vi "AutoFileCreatorMain.vi"() -> ()   [LabVIEW 2019]
uses:
  Utils/FilePath.vi
  <vilib>/Utility/inputDevices.llb/mouseAcquire.vi
  <vilib>/xml/NI_XML.lvlib
  <resource>/objmgr/DOMUserDefRef.rc
  <vilib>/FTP/NI_FTP.lvlib
panel:
  out "File Transfer Status":errorcluster
  in  "CopiedData":string
  in  "LocalFileNames":string[](array[string])=["1A.txt", "1B.txt", "1C.txt", "1D.txt", "2A.txt", "2B.txt", "2C.txt", "2D.txt", "3A.txt", "3B.txt", "3C.txt", "3D.txt", "4A.txt", "4B.txt", "4C.txt", "4D.txt"]
  out "standard output":string
  out "standard error":string="NI Linux Real-Time (run mode)\n\nLog in with your NI-Auth credentials.\n\n"
  in  "LocalFiles":i32(listbox)=2
  in  "SaveToLocal":bool
  in  "LoadFromLocal":bool
  in  "ExportToRobot":bool
  out "XML With IDs":string="<Sequential ID=\"1\">\n</Sequential>"
  in  "Commands":i32(listbox)=-1
  out "XML":string="<Sequential>\n</Sequential>"
  # "Instructions:\nSelect a command or structure element (Sequential, Parallel) from the Commands box and click in the XML box to the right of a \">\" to place it. \n\nAll elements in a sequential block will be executed in sequence, and those in a parallel block will be executed at the same time. You can nest these structure blocks inside themselves along with commands for complex behavior.\n\nClick ESC to unselect the current command selection.\n\nDouble click to open the options menu. Most of these options work on a specific element, but for these you do not have to click to the right of a \">\",  you can click in the element.\n\nThe Commands box is autopopulated from the VIs you put into the CommandTemplates folder in the Robot Project.\n\nYou can select a file in the LocalFiles box and load it into the editor or export it to the robot. Save your file with the save button. Make sure to save before exporting to the robot, as it exports what is saved not what is currently in the editor.\n\nNot yet implemented: Press Z to undo"
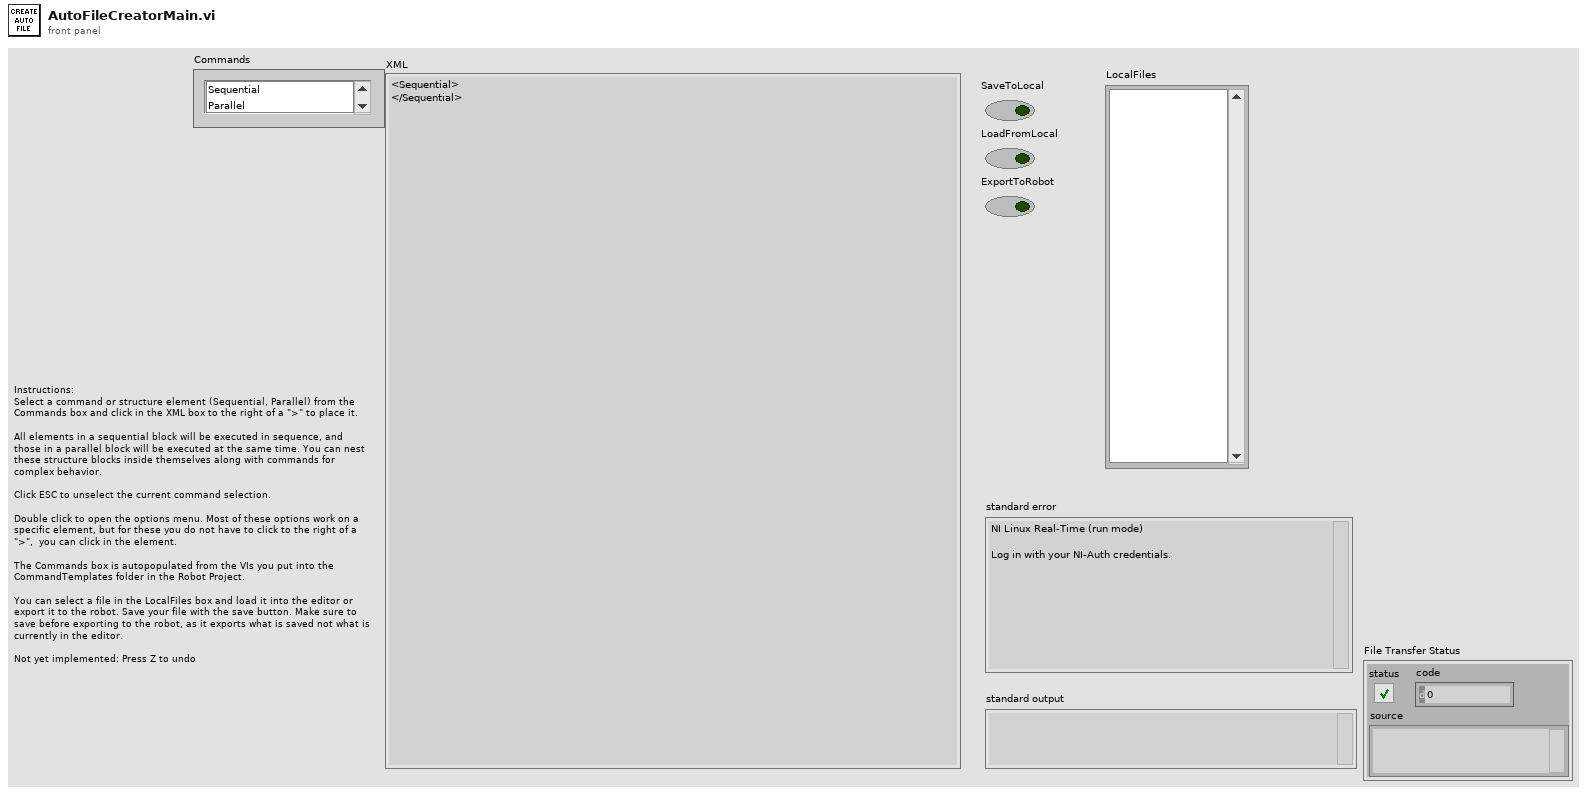
[diagram p1: front panel]
types:
  T1 = cluster{"Horizontal":i32, "Vertical":i32, "Scrolling":i32}
  T2 = typedef "eventvkey.ctl" = enum16{"ASCII", "Enter", "Return", "Shift", "Ctrl", "Alt", "Cmd", "Opt", "Caps", "NumLock", "Clear", "Break", "Up", "Down", "Left", "Right", "Insert", "Delete", "Home", "End", "PageUp", "PageDown", "Escape", "Help", "Pause", "ScrollLock", "F1", "F2", "F3", "F4", "F5", "F6", "F7", "F8", "F9", "F10", "F11", "F12", "F13", "F14", "F15", "F16", "F17", "F18", "F19", "F20", "F21", "F22", "F23", "F24", "Play", "VolumeUp", "VolumeDown", "Mute", "Two Byte Char"}
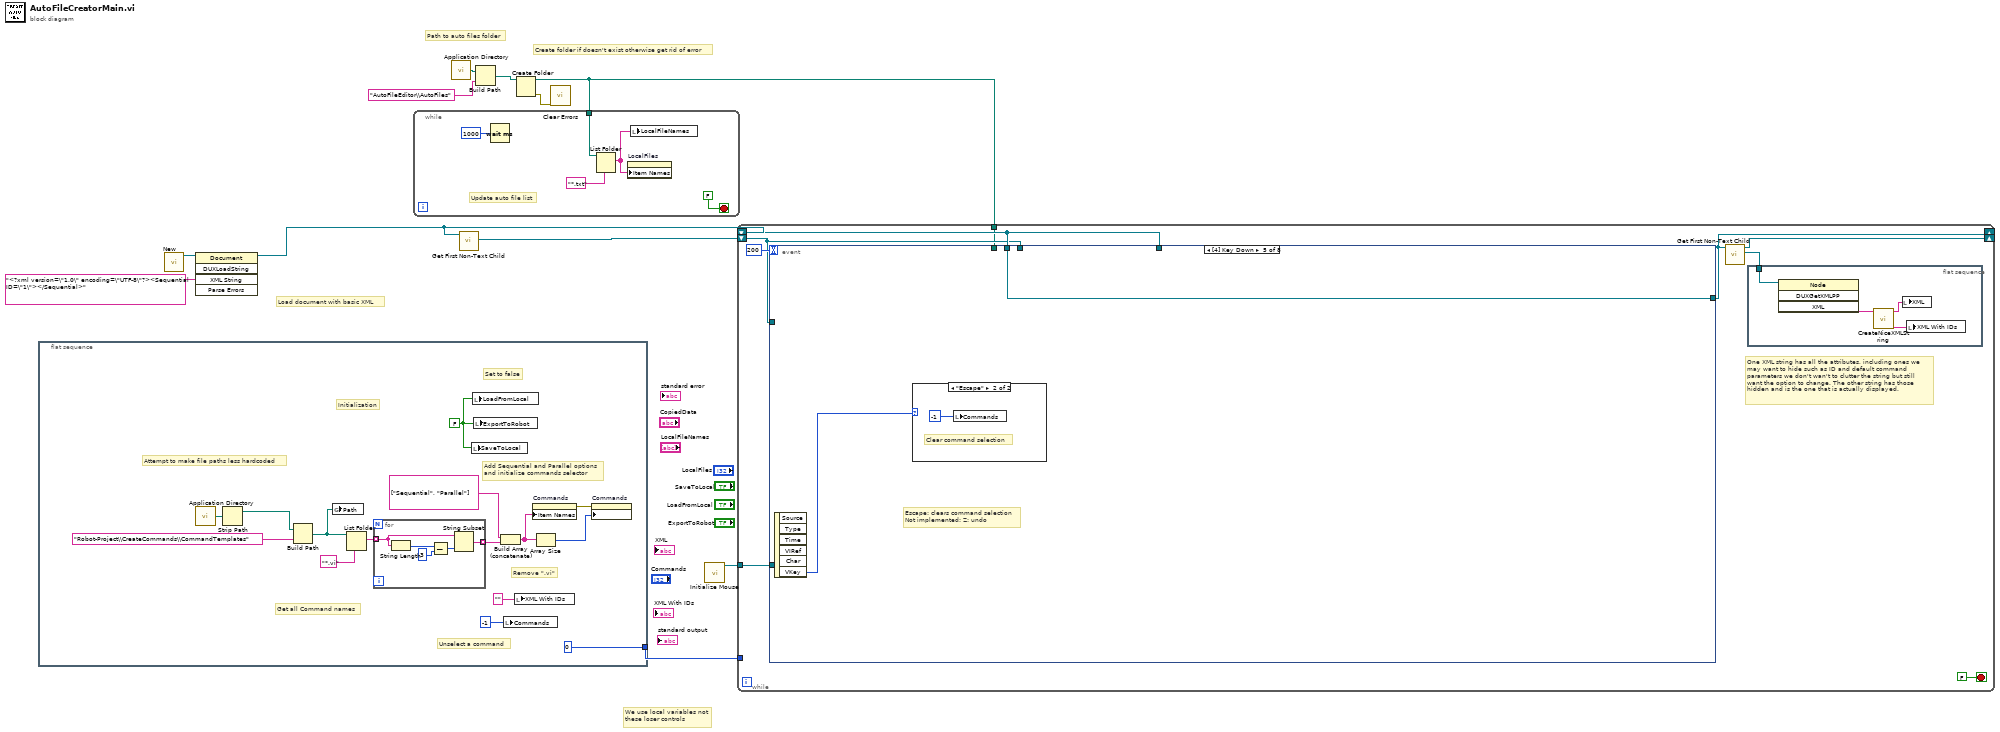
[diagram p0: block diagram]
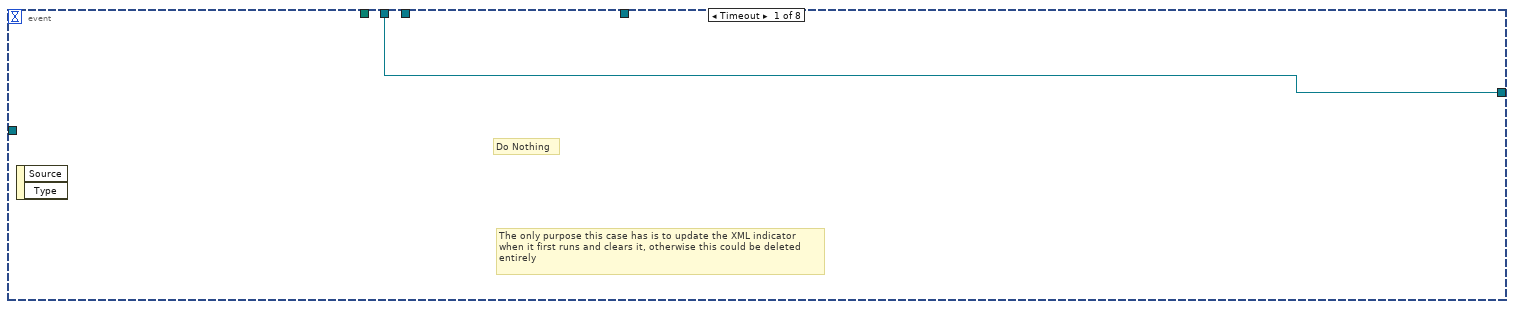
[diagram p2: hidden frame]
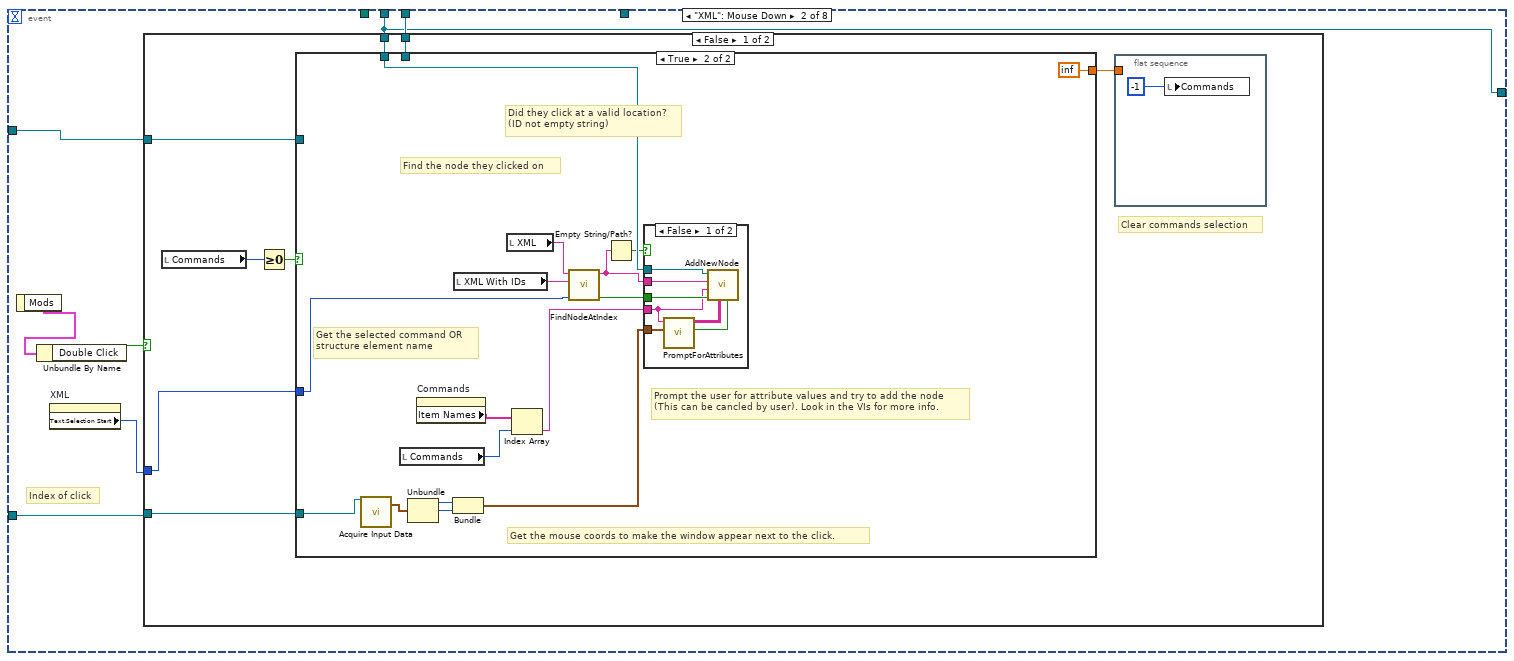
[diagram p3: hidden frame]
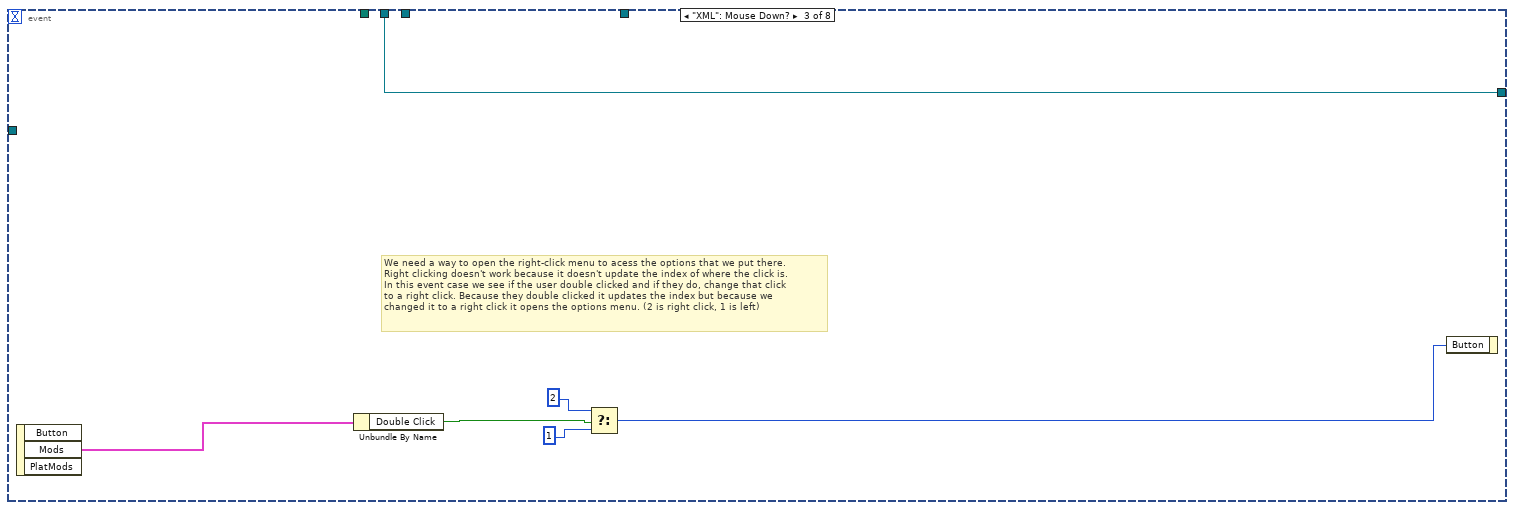
[diagram p7: hidden frame]
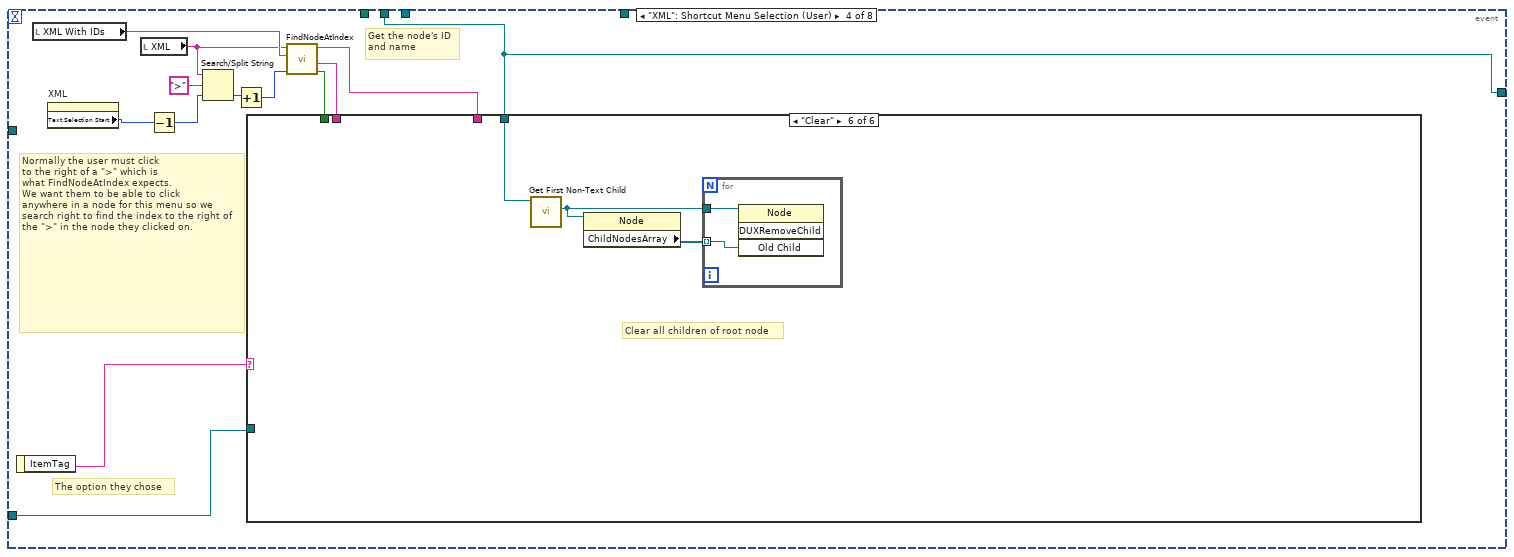
[diagram p8: hidden frame]
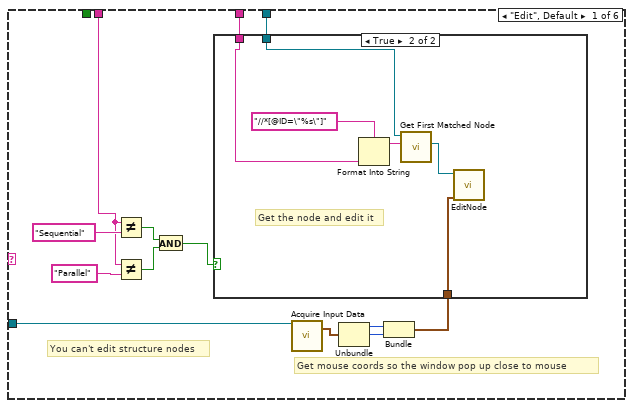
[diagram p9: hidden frame]
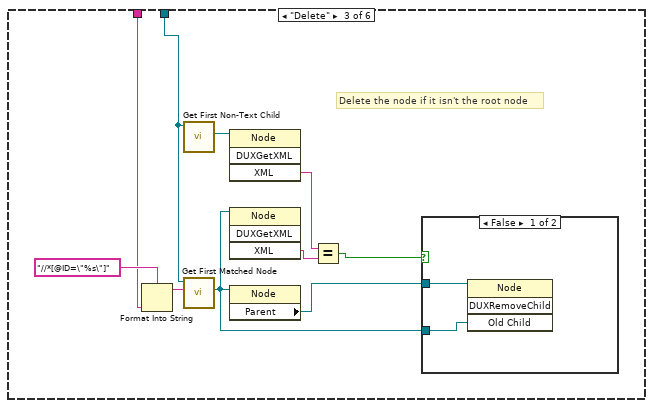
[diagram p12: hidden frame]
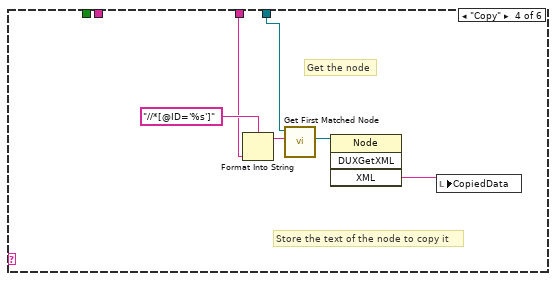
[diagram p14: hidden frame]
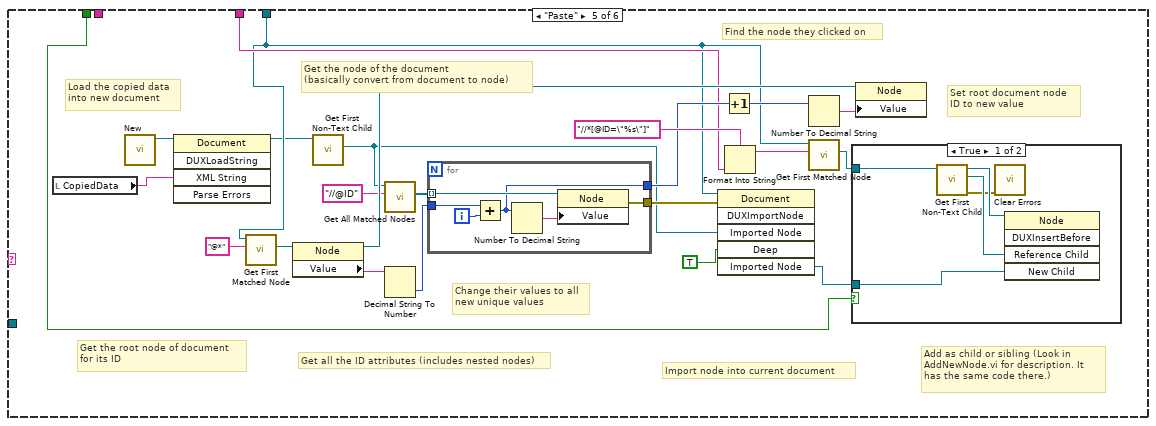
[diagram p15: hidden frame]
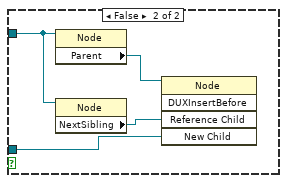
[diagram p16: hidden frame]
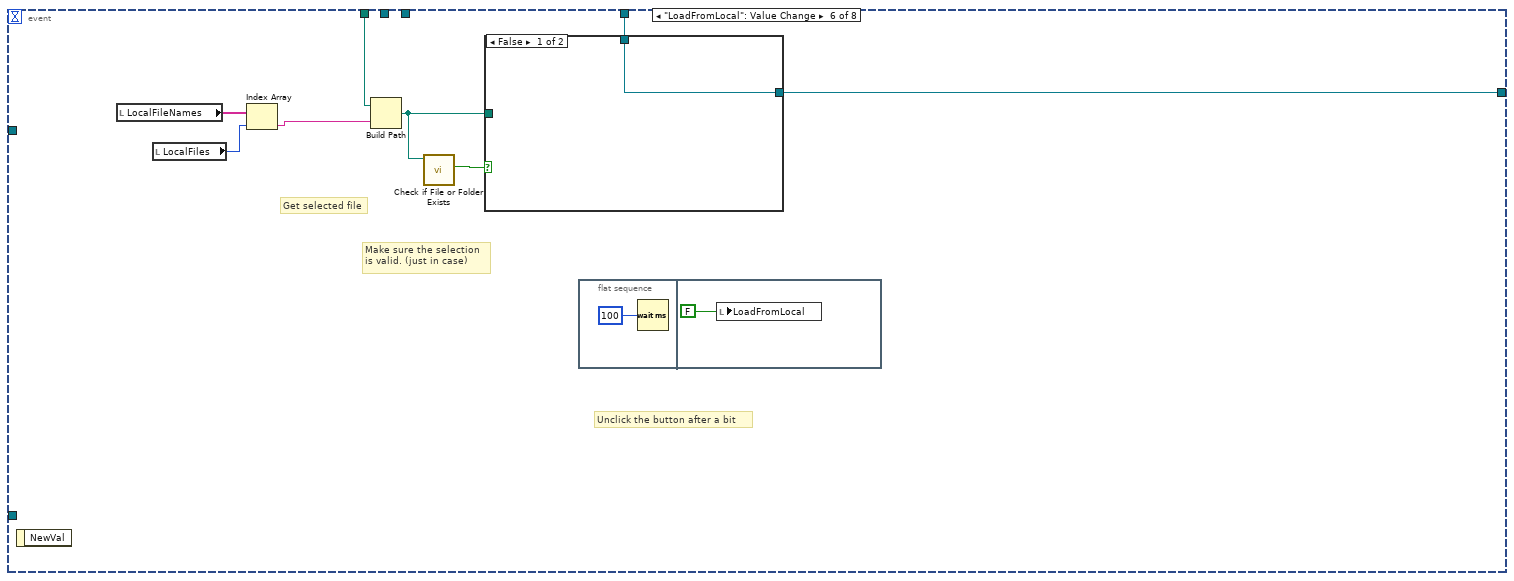
[diagram p18: hidden frame]
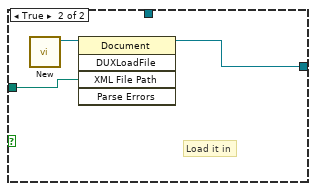
[diagram p19: hidden frame]
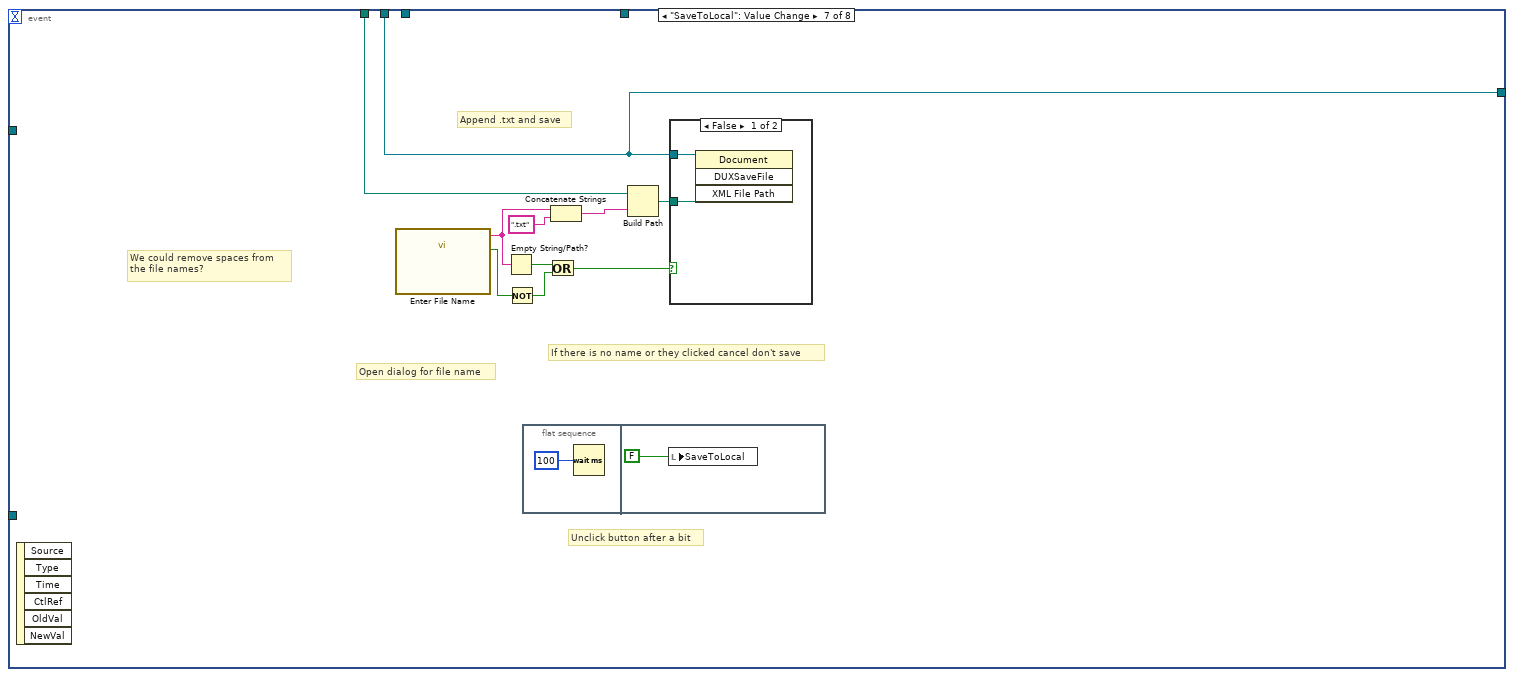
[diagram p20: hidden frame]
diagram:
  # "We use local variables not\nthese loser controls"
  # "Load document with basic XML"
  # "Create folder if doesn't exist otherwise get rid of error"
  # "Path to auto files folder"
  n1 = flat-sequence {
    tunnel: [0] -> w11
    frame #0 {
      w15 = FALSE ("SaveToLocal")
      # "Add Sequential and Parallel options\nand initialize commands selector"
      # "Remove \".vi\""
      # "Get all Command names"
      # "Attempt to make file paths less hardcoded"
      # "Unselect a command"
      # "Set to false"
      # "Initialization"
      n2 = call <vilib>:"Application Directory.vi"() -> ("Application Directory"=w12:path)
      n3 = Strip Path(path=w12) -> (stripped path=w14:path)  [unwired: 1 out]
      n4 = Build Path(base path=w14, name or relative path="Robot-Project\\CreateCommands\\CommandTemplates") -> (appended path=w13:path)
      n5 = global write "FilePath.vi" "Path"(w13) -> ()
      n6 = List Folder(path=w13, pattern="*.vi") -> (filenames=w19:string[])  [unwired: 2 in, 3 out]
      n7 = for {
        tunnel: w19 -> [w31] mode=indexing
        tunnel: [w27] -> w20 mode=indexing
        n8 = String Length(string=w31) -> (length=w30:i32)
        n9 = Subtract(x=w30, y=3) -> (x-y=w28:i32)
        n10 = String Subset(string=w31, length (rest)=w28) -> (substring=w27:string)  [unwired: 1 in]
      }
      n11 = local write "SaveToLocal"(w15) -> ()
      n12 = local write "LoadFromLocal"(w15) -> ()
      n13 = local write "ExportToRobot"(w15) -> ()
      n14 = Build Array (concatenate)(string[] ["Sequential", "Parallel"], w20) -> (w21:string[])
      n15 = local write "Commands"(-1 ("Active Row:Active Row Number")) -> ()
      n16 = local write "XML With IDs"("" ("XML With IDs")) -> ()
      n17 = property on="Commands" class="LstBox (strict)"("Item Names"=w21) -> (error out=w23:errorcluster)  [unwired: 2 in, 1 out]
      n18 = Array Size(array=w21) -> (size(s)=w22:i32)
      n19 = property on="Commands" class="LstBox (strict)"(error in=w23, "Number of Rows"=w22) -> ()  [unwired: 1 in, 2 out]
    }
  }
  n20 = call <vilib>:"New.vi"() -> ("DOM document out"=w10:refnum<k20>)  [unwired: 8 in, 1 out]
  n21 = invoke class="Document" method="DUXLoadString"(reference=w10, "XML String"="<?xml version=\"1.0\" encoding=\"UTF-8\"?><Sequential ID=\"1\"></Sequential>") -> (reference out=w9:refnum<k20>)  [unwired: 3 in, 4 out]
  n22 = call <vilib>:"Application Directory.vi"() -> ("Application Directory"=w4:path)
  n23 = call <vilib>:"Get First Non-Text Child.vi"("node in"=w9) -> ("child node"=w8:refnum<k20>)  [unwired: 7 in, 3 out]
  n24 = Build Path(base path=w4, name or relative path="AutoFileEditor\\AutoFiles") -> (appended path=w1:path)
  n25 = Create Folder(path (use dialog)=w1) -> (created path=w3:path, error out=w2:errorcluster)  [unwired: 2 in, 1 out]
  n26 = while {
    tunnel: w3 -> [w32]
    stop <- FALSE stop-if-true
    # "Update auto file list"
    n27 = Wait (ms)(milliseconds to wait=u32 1000) -> ()  [unwired: 1 out]
    n28 = List Folder(path=w32, pattern="*.txt") -> (filenames=w33:string[])  [unwired: 2 in, 3 out]
    n29 = property on="LocalFiles" class="LstBox (strict)"("Item Names"=w33) -> ()  [unwired: 2 in, 2 out]
    n30 = local write "LocalFileNames"(w33) -> ()
  }
  n31 = call <vilib>:"Clear Errors.vi"("error in (no error)"=w2) -> ()  [unwired: 5 in, 2 out]
  n32 = call <vilib>:"Initialize Mouse.vi"() -> ("device ID"=w7:refnum<k1>)  [unwired: 10 in, 1 out]
  n33 = while {
    tunnel: w11 -> [_]
    shift-right: [w38] -> _
    shift-left: w9 -> [w42]
    shift-right: [w40] -> _
    shift-left: w8 -> [w41]
    tunnel: w7 -> [w43]
    tunnel: w3 -> [w37]
    stop <- FALSE stop-if-true
    # "One XML string has all the attributes, including ones we\nmay want to hide such as ID and default command\nparameters we don't wan't to clutter the string but still\nwant the option to change. The other string has those\nhidden and is the one that is actually displayed."
    n34 = event shown="[4] Key Down" {
      selector: _ -> [_ _ _ _ _ _ _ _]
      dyn-events: _ -> [_ _ _ _ _ _ _ _]
      timeout: 200 -> [_ _ _ _ _ _ _ _]
      tunnel: w41 -> [_ w57 _ _ _ _ _ _]
      tunnel: w42 -> [w50 w51 w90 w98 w189 _ w207 w221]
      tunnel: w41 -> [_ w56 _ _ _ _ _ _]
      tunnel: w43 -> [_ w55 _ w96 _ _ _ _]
      tunnel: w42 -> [_ _ _ _ _ w192 _ _]
      tunnel: [w50 w51 w90 w98 w189 w198 w207 w221] -> w38
      tunnel: w37 -> [_ _ _ _ _ w196 w206 w220]
      event Timeout {
        # "The only purpose this case has is to update the XML indicator\nwhen it first runs and clears it, otherwise this could be deleted\nentirely"
        # "Do Nothing"
        n35 = event-data() -> ()  [unwired: 1 in, 2 out]
      }
      event "XML": Mouse Down {
        # "Index of click"
        n36 = event-data() -> ("Mods"=w54:cluster{"Double Click":bool, "Menu Key":bool})  [unwired: 1 in]
        n37 = Unbundle By Name(w54) -> ("Double Click"=w53:bool)
        n38 = property on="XML" class="Str"() -> ("Text.Selection Start"=w52:u32)  [unwired: 2 in, 2 out]
        n39 = case shown="False" w53 {
          tunnel: w57 -> [w63 _]
          tunnel: w51 -> [w62 _]
          tunnel: w56 -> [w61 _]
          tunnel: w55 -> [w59 _]
          tunnel: w52 -> [w58 _]
          frame False {
            # "Clear commands selection"
            n40 = local read "Commands"() -> (w65:i32)
            n41 = Greater Or Equal To 0?(x=w65) -> (x >= 0?=w64:bool)
            n42 = case shown="True" w64 {
              tunnel: w63 -> [_ _]
              tunnel: w62 -> [_ w74]
              tunnel: w61 -> [_ _]
              tunnel: w58 -> [_ w78]
              tunnel: [_ inf] -> w60
              tunnel: w59 -> [_ w72]
              frame False {
                # "If no command is selected do nothing"
              }
              frame True {
                # "Prompt the user for attribute values and try to add the node\n(This can be cancled by user). Look in the VIs for more info."
                # "Did they click at a valid location?\n(ID not empty string)"
                # "Find the node they clicked on"
                # "Get the selected command OR\nstructure element name"
                # "Get the mouse coords to make the window appear next to the click."
                n43 = call-poly <vilib>:"Acquire Input Data.vi"("device ID"=w72) -> ("axis info"=w71:T1)  [unwired: 15 in, 3 out]
                n44 = local read "Commands"() -> (w80:i32)
                n45 = Unbundle(w71) -> ("Horizontal"=w70:i32, "Vertical"=w69:i32)  [unwired: 1 out]
                n46 = property on="Commands" class="LstBox (strict)"() -> ("Item Names"=w81:string[])  [unwired: 2 in, 2 out]
                n47 = Bundle("Horizontal"=w70, "Vertical"=w69) -> (w66:cluster{"Horizontal":i32, "Vertical":i32})  [unwired: 1 in]
                n48 = local read "XML With IDs"() -> (w77:string)
                n49 = local read "XML"() -> (w76:string)
                n50 = Index Array(array=w81, index=w80) -> (element=w73:string)
                n51 = call "FindNodeAtIndex.vi"("ClickIndex"=w78, "XML with IDs"=w77, "XML In"=w76) -> ("Insert as child not sibling"=w75:bool, "Node ID"=w68:string)  [unwired: 6 in, 1 out]
                n52 = Empty String/Path?(string/path=w68) -> (empty?=w67:bool)
                n53 = case shown="False" w67 {
                  tunnel: w75 -> [w88 _]
                  tunnel: w74 -> [w87 _]
                  tunnel: w73 -> [w84 _]
                  tunnel: w68 -> [w86 _]
                  tunnel: w66 -> [w85 _]
                  frame False {
                    n54 = call "PromptForAttributes.vi"("Mouse Coords"=w85, "New Node Name"=w84) -> ("Canceled"=w83:bool, "Attributes"=w82:string[][])  [unwired: 8 in]
                    n55 = call "AddNewNode.vi"("Cancel"=w83, "Attributes"=w82, "Insert As Child"=w88, "New Node Name"=w84, "Node ID"=w86, "DOM document"=w87) -> ()  [unwired: 6 in]
                  }
                  frame True {
                  }
                }
              }
            }
            n56 = flat-sequence {
              tunnel: w60 -> [_]
              frame #0 {
                n57 = local write "Commands"(-1 ("Active Row:Active Row Number")) -> ()
              }
            }
          }
          frame True {
            # "Leave double clicking to the other event case"
          }
        }
      }
      event "XML": Mouse Down? {
        # "We need a way to open the right-click menu to acess the options that we put there.\nRight clicking doesn't work because it doesn't update the index of where the click is.\nIn this event case we see if the user double clicked and if they do, change that click\nto a right click. Because they double clicked it updates the index but because we\nchanged it to a right click it opens the options menu. (2 is right click, 1 is left)"
        n58 = event-data() -> ("Mods"=w95:cluster{"Double Click":bool, "Menu Key":bool})  [unwired: 1 in, 2 out]
        n59 = Unbundle By Name(w95) -> ("Double Click"=w94:bool)
        n60 = Select(t=u16 2 ("Button"), s=w94, f=u16 1 ("Button")) -> (s? t:f=w91:u16)
        n61 = event-data("Button"=w91) -> ()  [unwired: 1 in, 1 out]
      }
      event "XML": Shortcut Menu Selection (User) {
        # "Normally the user must click\nto the right of a \">\" which is\nwhat FindNodeAtIndex expects.\nWe want them to be able to click\nanywhere in a node for this menu so we search right to find the index to the right of the \">\" in the node they clicked on."
        # "The option they chose"
        # "Get the node's ID\nand name"
        n62 = event-data() -> ("ItemTag"=w103:string)  [unwired: 1 in]
        n63 = local read "XML With IDs"() -> (w100:string)
        n64 = property on="XML" class="Str"() -> ("Text.Selection Start"=w108:u32)  [unwired: 2 in, 2 out]
        n65 = local read "XML"() -> (w99:string)
        n66 = Decrement(x=w108) -> (x-1=w106:u32)
        n67 = Search/Split String(string=w99, search string/char (-)=">", offset (0)=w106) -> (offset of match=w104:i32)  [unwired: 2 out]
        n68 = Increment(x=w104) -> (x+1=w105:i32)
        n69 = call "FindNodeAtIndex.vi"("ClickIndex"=w105, "XML with IDs"=w100, "XML In"=w99) -> ("Insert as child not sibling"=w97:bool, "Node Name"=w101:string, "Node ID"=w102:string)  [unwired: 6 in]
        n70 = case shown="\"Clear\"" w103 {
          tunnel: w102 -> [w121 _ w135 w141 w148 _]
          tunnel: w98 -> [w120 _ w128 w142 w147 w186]
          tunnel: w101 -> [w117 _ _ _ _ _]
          tunnel: w97 -> [_ _ _ _ w149 _]
          tunnel: w96 -> [w110 _ _ _ _ _]
          frame "Edit", Default {
            # "Get mouse coords so the window pop up close to mouse"
            # "You can't edit structure nodes"
            n71 = Not Equal?(x=w117, y="Sequential") -> (x != y?=w118:bool)
            n72 = Not Equal?(x=w117, y="Parallel") -> (x != y?=w115:bool)
            n73 = And(x=w118, y=w115) -> (x .and. y?=w114:bool)
            n74 = call-poly <vilib>:"Acquire Input Data.vi"("device ID"=w110) -> ("axis info"=w113:T1)  [unwired: 15 in, 3 out]
            n75 = Unbundle(w113) -> ("Horizontal"=w112:i32, "Vertical"=w111:i32)  [unwired: 1 out]
            n76 = Bundle("Horizontal"=w112, "Vertical"=w111) -> (w109:cluster{"Horizontal":i32, "Vertical":i32})  [unwired: 1 in]
            n77 = case shown="True" w114 {
              tunnel: w121 -> [_ w125]
              tunnel: w120 -> [_ w123]
              tunnel: w109 -> [_ w122]
              frame False {
              }
              frame True {
                # "Get the node and edit it"
                n78 = Format Into String(format string="//*[@ID=\"%s\"]", w125) -> (resulting string=w127:string)  [unwired: 2 in, 1 out]
                n79 = call <vilib>:"Get First Matched Node.vi"("XPath expression"=w127, "node in"=w123) -> ("node result"=w124:refnum<k20>)  [unwired: 7 in, 2 out]
                n80 = call "EditNode.vi"("Mouse Coords"=w122, "Node"=w124) -> ()  [unwired: 10 in]
              }
            }
          }
          frame "Move" {
            # "Not implemented yet"
          }
          frame "Delete" {
            # "Delete the node if it isn't the root node"
            n81 = Format Into String(format string="//*[@ID=\"%s\"]", w135) -> (resulting string=w137:string)  [unwired: 2 in, 1 out]
            n82 = call <vilib>:"Get First Non-Text Child.vi"("node in"=w128) -> ("child node"=w133:refnum<k20>)  [unwired: 7 in, 3 out]
            n83 = call <vilib>:"Get First Matched Node.vi"("XPath expression"=w137, "node in"=w128) -> ("node result"=w131:refnum<k20>)  [unwired: 7 in, 2 out]
            n84 = invoke class="Node" method="DUXGetXML"(reference=w133) -> ("XML"=w132:string)  [unwired: 3 in, 3 out]
            n85 = invoke class="Node" method="DUXGetXML"(reference=w131) -> ("XML"=w130:string)  [unwired: 3 in, 3 out]
            n86 = property class="Node"(reference=w131) -> ("Parent"=w134:refnum<k20>)  [unwired: 1 in, 2 out]
            n87 = Equal?(x=w132, y=w130) -> (x = y?=w129:bool)
            n88 = case shown="False" w129 {
              tunnel: w134 -> [w139 _]
              tunnel: w131 -> [w138 _]
              frame False {
                n89 = invoke class="Node" method="DUXRemoveChild"(reference=w139, "Old Child"=w138) -> ()  [unwired: 2 in, 4 out]
              }
              frame True {
              }
            }
          }
          frame "Copy" {
            # "Get the node"
            # "Store the text of the node to copy it"
            n90 = Format Into String(format string="//*[@ID='%s']", w141) -> (resulting string=w144:string)  [unwired: 2 in, 1 out]
            n91 = call <vilib>:"Get First Matched Node.vi"("XPath expression"=w144, "node in"=w142) -> ("node result"=w143:refnum<k20>)  [unwired: 7 in, 2 out]
            n92 = invoke class="Node" method="DUXGetXML"(reference=w143) -> ("XML"=w140:string)  [unwired: 3 in, 3 out]
            n93 = local write "CopiedData"(w140) -> ()
          }
          frame "Paste" {
            # "Add as child or sibling (Look in\nAddNewNode.vi for description. It\nhas the same code there.)"
            # "Import node into current document"
            # "Find the node they clicked on"
            # "Get the node of the document\n(basically convert from document to node)"
            # "Set root document node\nID to new value"
            # "Change their values to all\nnew unique values"
            # "Get all the ID attributes (includes nested nodes)"
            # "Get the root node of document\nfor its ID"
            # "Load the copied data\ninto new document"
            n94 = local read "CopiedData"() -> (w150:string)
            n95 = call <vilib>:"New.vi"() -> ("DOM document out"=w168:refnum<k20>)  [unwired: 8 in, 1 out]
            n96 = invoke class="Document" method="DUXLoadString"(reference=w168, "XML String"=w150) -> (reference out=w146:refnum<k20>)  [unwired: 3 in, 4 out]
            n97 = call <vilib>:"Get First Matched Node.vi"("XPath expression"="@*", "node in"=w147) -> ("node result"=w163:refnum<k20>)  [unwired: 7 in, 2 out]
            n98 = property class="Node"(reference=w163) -> (reference out=w159:refnum<k20>, "Value"=w161:string)  [unwired: 1 in, 1 out]
            n99 = call <vilib>:"Get First Non-Text Child.vi"("node in"=w146) -> ("child node"=w151:refnum<k20>)  [unwired: 7 in, 3 out]
            n100 = call <vilib>:"Get All Matched Nodes.vi"("XPath expression"="//@ID", "node in"=w151) -> ("node result array"=w156:refnum<k20>[])  [unwired: 7 in, 2 out]
            n101 = Decimal String To Number(string=w161) -> (number=w153:i32)  [unwired: 2 in, 1 out]
            n102 = for {
              tunnel: w156 -> [w174] mode=indexing
              tunnel: [w172] -> w155
              tunnel: w153 -> [w170]
              tunnel: [w169] -> w152
              i -> [w173]
              n103 = Add(x=w170, y=w173) -> (x+y=w172:i32)
              n104 = Number To Decimal String(number=w172) -> (decimal integer string=w171:string)  [unwired: 1 in]
              n105 = property class="Node"(reference=w174, "Value"=w171) -> (error out=w169:errorcluster)  [unwired: 1 in, 1 out]
            }
            n106 = invoke class="Document" method="DUXImportNode"(reference=w147, error in=w152, "Imported Node"=w151, "Deep"=TRUE) -> ("Imported Node"=w158:refnum<k20>)  [unwired: 2 in, 5 out]
            n107 = Increment(x=w155) -> (x+1=w154:i32)
            n108 = Format Into String(format string="//*[@ID=\"%s\"]", w148) -> (resulting string=w166:string)  [unwired: 2 in, 1 out]
            n109 = Number To Decimal String(number=w154) -> (decimal integer string=w160:string)  [unwired: 1 in]
            n110 = call <vilib>:"Get First Matched Node.vi"("XPath expression"=w166, "node in"=w147) -> ("node result"=w165:refnum<k20>)  [unwired: 7 in, 2 out]
            n111 = case shown="True" w149 {
              tunnel: w165 -> [w176 w182]
              tunnel: w158 -> [w175 w180]
              frame True {
                n112 = call <vilib>:"Get First Non-Text Child.vi"("node in"=w176) -> ("error out"=w177:errorcluster, "child node"=w178:refnum<k20>, "node out"=w179:refnum<k20>)  [unwired: 7 in, 1 out]
                n113 = call <vilib>:"Clear Errors.vi"("error in (no error)"=w177) -> ()  [unwired: 5 in, 2 out]
                n114 = invoke class="Node" method="DUXInsertBefore"(reference=w179, "Reference Child"=w178, "New Child"=w175) -> ()  [unwired: 2 in, 5 out]
              }
              frame False {
                n115 = property class="Node"(reference=w182) -> ("Parent"=w181:refnum<k20>)  [unwired: 1 in, 2 out]
                n116 = property class="Node"(reference=w182) -> ("NextSibling"=w183:refnum<k20>)  [unwired: 1 in, 2 out]
                n117 = invoke class="Node" method="DUXInsertBefore"(reference=w181, "Reference Child"=w183, "New Child"=w180) -> ()  [unwired: 2 in, 5 out]
              }
            }
            n118 = property class="Node"(reference=w159, "Value"=w160) -> ()  [unwired: 1 in, 2 out]
          }
          frame "Clear" {
            # "Clear all children of root node"
            n119 = call <vilib>:"Get First Non-Text Child.vi"("node in"=w186) -> ("child node"=w184:refnum<k20>)  [unwired: 7 in, 3 out]
            n120 = property class="Node"(reference=w184) -> ("ChildNodesArray"=w185:refnum<k20>[])  [unwired: 1 in, 2 out]
            n121 = for {
              tunnel: w184 -> [w188]
              tunnel: w185 -> [w187] mode=indexing
              n122 = invoke class="Node" method="DUXRemoveChild"(reference=w188, "Old Child"=w187) -> ()  [unwired: 2 in, 4 out]
            }
          }
        }
      }
      event Key Down {
        # "Escape: clears command selection\nNot implemented: Z: undo"
        n123 = event-data() -> ("VKey"=w190:T2)  [unwired: 1 in, 5 out]
        n124 = case shown="\"Escape\"" w190 {
          frame "ASCII", Default {
          }
          frame "Escape" {
            # "Clear command selection"
            n125 = local write "Commands"(-1 ("Active Row:Active Row Number")) -> ()
          }
        }
      }
      event "LoadFromLocal": Value Change {
        # "Make sure the selection\nis valid. (just in case)"
        # "Get selected file"
        # "Unclick the button after a bit"
        n126 = event-data() -> ()  [unwired: 1 in, 1 out]
        n127 = local read "LocalFileNames"() -> (w199:string[])
        n128 = local read "LocalFiles"() -> (w195:i32)
        n129 = Index Array(array=w199, index=w195) -> (element=w197:string)
        n130 = Build Path(base path=w196, name or relative path=w197) -> (appended path=w194:path)
        n131 = call <vilib>:"Check if File or Folder Exists.vi"("path"=w194) -> ("file or folder exists?"=w193:bool)  [unwired: 8 in, 2 out]
        n132 = case shown="False" w193 {
          tunnel: [w200 w202] -> w198
          tunnel: w194 -> [_ w201]
          tunnel: w192 -> [w200 _]
          frame False {
          }
          frame True {
            # "Load it in"
            n133 = call <vilib>:"New.vi"() -> ("DOM document out"=w203:refnum<k20>)  [unwired: 8 in, 1 out]
            n134 = invoke class="Document" method="DUXLoadFile"(reference=w203, "XML File Path"=w201) -> (reference out=w202:refnum<k20>)  [unwired: 3 in, 4 out]
          }
        }
        n135 = flat-sequence {
          frame #0 {
            n136 = Wait (ms)(milliseconds to wait=u32 100) -> ()  [unwired: 1 out]
          }
          frame #1 {
            n137 = local write "LoadFromLocal"(FALSE ("SaveToLocal")) -> ()
          }
        }
      }
      event "SaveToLocal": Value Change {
        # "We could remove spaces from\nthe file names?"
        # "Append .txt and save"
        # "If there is no name or they clicked cancel don't save"
        # "Open dialog for file name"
        # "Unclick button after a bit"
        n138 = event-data() -> ()  [unwired: 1 in, 6 out]
        n139 = call "Enter File Name"() -> ("File Name"=w209:string, "Enter"=w213:bool)  [unwired: 17 in, 1 out]
        n140 = Empty String/Path?(string/path=w209) -> (empty?=w215:bool)
        n141 = Not(x=w213) -> (.not. x?=w214:bool)
        n142 = flat-sequence {
          frame #0 {
            n143 = Wait (ms)(milliseconds to wait=u32 100) -> ()  [unwired: 1 out]
          }
          frame #1 {
            n144 = local write "SaveToLocal"(FALSE ("SaveToLocal")) -> ()
          }
        }
        n145 = Or(x=w215, y=w214) -> (x .or. y?=w208:bool)
        n146 = Concatenate Strings(w209, ".txt" ("string")) -> (w211:string)
        n147 = Build Path(base path=w206, name or relative path=w211) -> (appended path=w210:path)
        n148 = case shown="False" w208 {
          tunnel: w207 -> [w217 _]
          tunnel: w210 -> [w216 _]
          frame False {
            n149 = invoke class="Document" method="DUXSaveFile"(reference=w217, "XML File Path"=w216) -> ()  [unwired: 2 in, 4 out]
          }
          frame True {
          }
        }
      }
      event "ExportToRobot": Value Change {
        # "Path to where file should go on robot"
        # "Call the command"
        # "Generate a string that will run in the terminal\nthat will call scp to export the file to the robot"
        # "Scp command"
        # "Get the file path"
        # "Unclick when done"
        # "replace backslash with slash\nand change begining to /c/"
        n150 = event-data() -> ()  [unwired: 1 in, 6 out]
        n151 = disable-structure shown="Disabled" {
          frame Disabled {
            n152 = call <vilib>:"FTP Put File.vi"("password"="", "user"="anonymous", "remote path"="/home/lvuser/Auto/AutoFiles/", "host"="lvuser@roborio-1712-frc.local") -> ("file error"=→"File Transfer Status":errorcluster)  [unwired: 6 in, 1 out]
          }
          frame Enabled {
          }
        }
        n153 = local read "LocalFileNames"() -> (w240:string[])
        n154 = local read "LocalFiles"() -> (w239:i32)
        n155 = Index Array(array=w240, index=w239) -> (element=w241:string)
        n156 = Build Path(base path=w220, name or relative path=w241) -> (appended path=w224:path)
        n157 = Path To String(path=w224) -> (string=w231:string)
        n158 = String Subset(string=w231, offset (0)=2) -> (substring=w229:string)  [unwired: 1 in]
        n159 = Search and Replace String(replace all?=TRUE ("replace all? (F)"), input string=w229, search string="\\", replace string="/" ("replace string (\"\")")) -> (result string=w228:string)  [unwired: 4 in, 3 out]
        n160 = Concatenate Strings("\"/c" ("string"), w228, "\"" ("string")) -> (w226:string)
        n161 = Concatenate Strings("\"C:\\Program Files\\Git\\usr\\bin\\scp.exe\" " ("command line"), w226, " lvuser@roboRIO-1712-FRC.local:/home/lvuser/Auto/AutoFiles/" ("string")) -> (w235:string)
        n162 = call <vilib>:"System Exec.vi"("wait until completion? (T)"=TRUE, "command line"=w235) -> ("standard error"=w222:string, "standard output"=w223:string)  [unwired: 6 in, 2 out]
        n163 = local write "standard error"(w222) -> ()
        n164 = flat-sequence {
          tunnel: w222 -> [_]
          frame #0 {
            n165 = local write "ExportToRobot"(FALSE ("ExportToRobot")) -> ()
          }
        }
        n166 = local write "standard output"(w223) -> ()
      }
    }
    n167 = call <vilib>:"Get First Non-Text Child.vi"("node in"=w38) -> ("child node"=w39:refnum<k20>, "node out"=w40:refnum<k20>)  [unwired: 7 in, 2 out]
    n168 = flat-sequence {
      tunnel: w39 -> [w46]
      frame #0 {
        n169 = invoke class="Node" method="DUXGetXMLPP"(reference=w46) -> ("XML"=w47:string)  [unwired: 3 in, 3 out]
        n170 = call "CreateNiceXMLString.vi"("XML In"=w47) -> ("XML String With IDs"=w48:string, "XML String Human Readable"=w49:string)  [unwired: 9 in]
        n171 = local write "XML"(w49) -> ()
        n172 = local write "XML With IDs"(w48) -> ()
      }
    }
  }
